vi "__READ_PM_1ch_E4419A_aveg.VI"(5 "aveg":i32=1, 6 "frq(GHz)":dbl=12.0, 7 "GPIB":string="13") -> (3 "chA":dbl=-19.9032016 format="%.4f")   [LabVIEW 2017]
panel:
  out "•¶Žš—ñ":string="-1.99032016E+001\n"
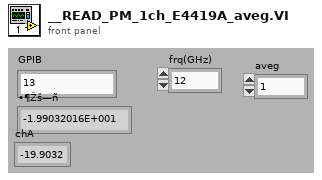
[diagram p1: front panel]
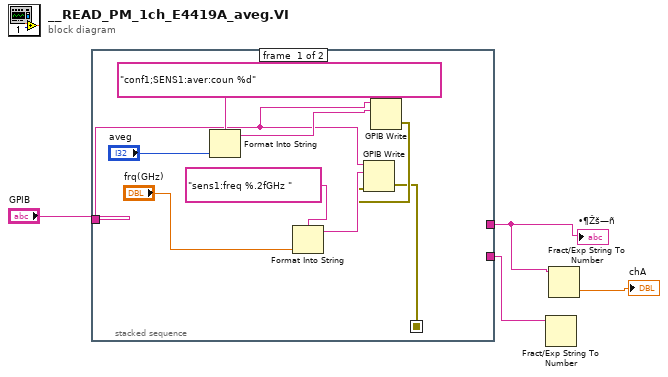
[diagram p0: block diagram]
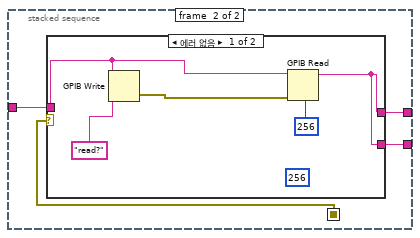
[diagram p2: hidden frame]
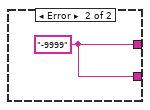
[diagram p3: hidden frame]
diagram:
  n1 = stacked-sequence {
    seq-local: [w5 _] -> [_ w14]
    tunnel: "GPIB" -> [w10 w17]
    tunnel: [_ w16] -> w3
    tunnel: [_ w15] -> w1
    frame #0 {
      n2 = Format Into String(format string="conf1;SENS1:aver:coun %d", "aveg") -> (resulting string=w11:string)  [unwired: 2 in, 1 out]
      n3 = Format Into String(format string="sens1:freq %.2fGHz ", "frq(GHz)") -> (resulting string=w7:string)  [unwired: 2 in, 1 out]
      n4 = GPIB Write(0:w10, 1:w11) -> (6:w6:errorcluster)  [unwired: 3 in, 1 out]
      n5 = GPIB Write(0:w10, 1:w7, 3:w6) -> (6:w5:errorcluster)  [unwired: 2 in, 1 out]
    }
    frame #1 {
      n6 = case shown="에러 없음" w14 {
        tunnel: w17 -> [w19 _]
        tunnel: [w18 w23] -> w16
        tunnel: [w18 w23] -> w15
        frame No Error {
          (unwired) 256
          n7 = GPIB Write(0:w19, 1:"read?") -> (6:w20:errorcluster)  [unwired: 3 in, 1 out]
          n8 = GPIB Read(0:w19, 1:256, 3:w20) -> (5:w18:string)  [unwired: 2 in, 2 out]
        }
        frame Error {
          w23 = "-9999"
        }
      }
    }
  }
  "•¶Žš—ñ" <- w3
  n9 = Fract/Exp String To Number(string=w1) -> ()  [unwired: 3 in, 2 out]
  n10 = Fract/Exp String To Number(string=w3) -> (number=→"chA":dbl)  [unwired: 3 in, 1 out]
